vi "force_control_loop_1axis.vi"(0 "Force In":dbl[](array[numeric]), 5 "Goal Position IN":dbl[][](array[numeric]), 7 "Force Stimulus":dbl[](array[numeric])) -> (6 "Force Position Out":dbl[](array[numeric]), 15 "Last Error":dbl[](array[numeric]))   [LabVIEW 2013]
uses:
  <vilib>/Analysis/NI_AALBase.lvlib
  <vilib>/Analysis/baseanly.llb/Real A x B.vi
  <vilib>/Analysis/Matrix/NI_Matrix.lvlib
  <vilib>/Analysis/Matrix/Numeric/Conversions/Matrix To Array - RM.vi
  force_control_globals.vi
  <vilib>/Analysis/Matrix/Datatypes/RealMatrix.ctl
panel:
  out "Goal Position HOLD":dbl[][](array[numeric])
  out "Last dForce":dbl[](array[numeric])
  out "Inject Stimulus":bool
  out "Last Force":dbl[](array[numeric])
  in  "Accel Transform":T1
  out "Last Ki":dbl[](array[numeric])
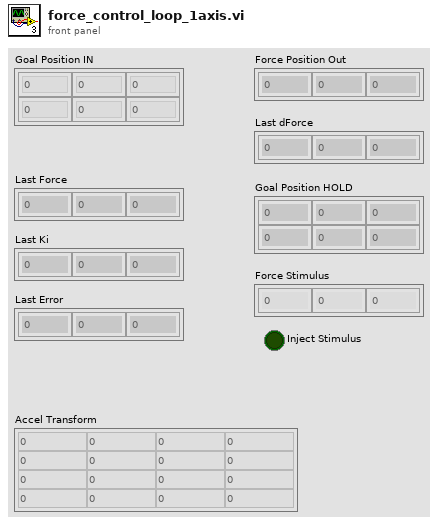
[diagram p1: front panel]
types:
  T1 = typedef "NI_Matrix.lvlib/RealMatrix.ctl" = dbl[][]
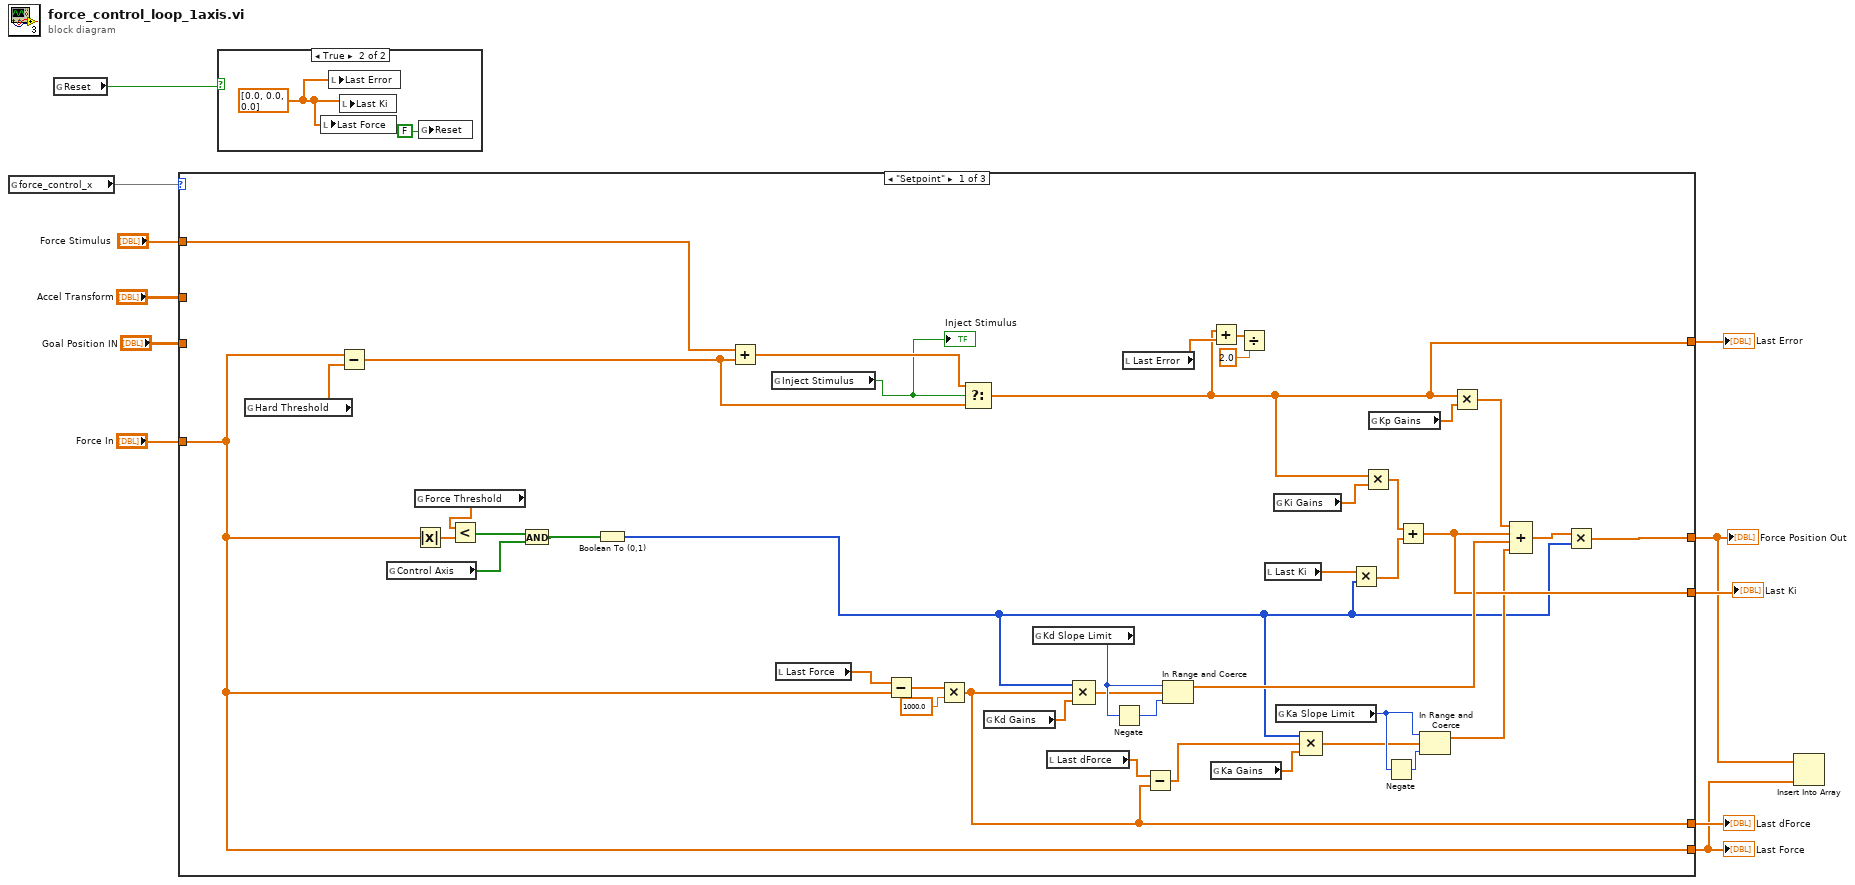
[diagram p0: block diagram]
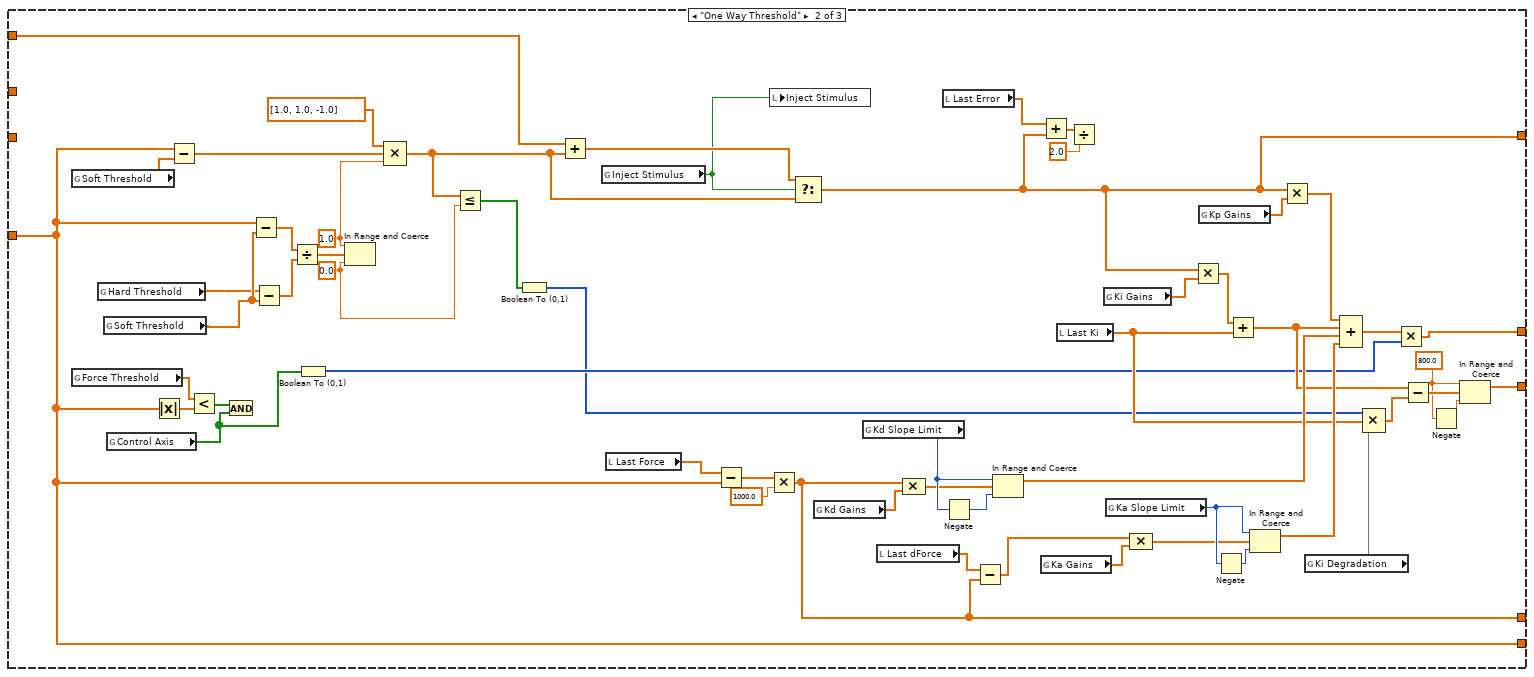
[diagram p3: hidden frame]
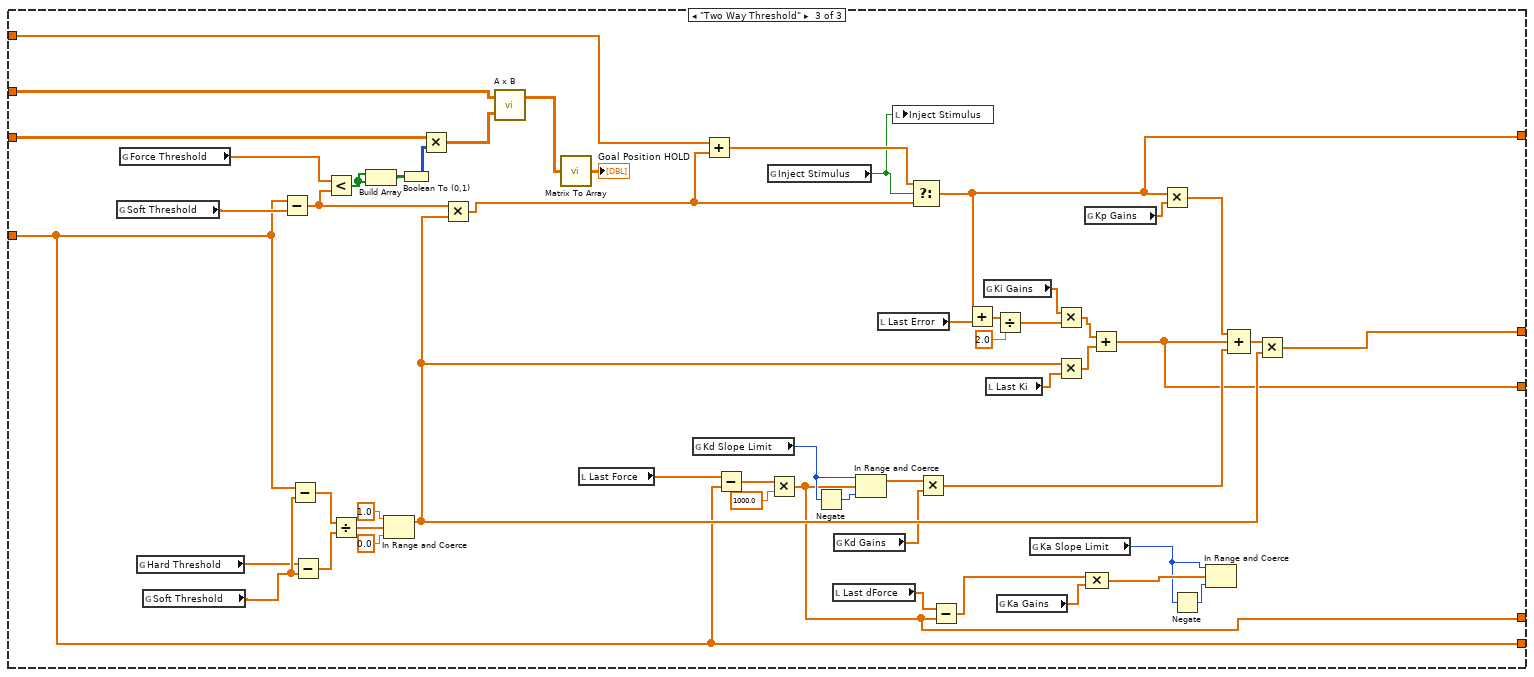
[diagram p4: hidden frame]
diagram:
  n1 = global read "force_control_globals.vi" "force_control_x"() -> (w10)
  n2 = global read "force_control_globals.vi" "Reset"() -> (w5:bool)
  n3 = case shown="\"Setpoint\"" w10 {
    tunnel: "Force In" -> [w34 w76 w112]
    tunnel: [w28 w57 w109] -> w4
    tunnel: [w27 w71 w147] -> w7
    tunnel: [w30 w59 w145] -> w2
    tunnel: "Accel Transform" -> [_ _ w132]
    tunnel: "Force Stimulus" -> [w41 w98 w120]
    tunnel: [w34 w76 w112] -> w1
    tunnel: "Goal Position IN" -> [_ _ w118]
    tunnel: [w22 w87 w111] -> w6
    frame "Setpoint" {
      n4 = global read "force_control_globals.vi" "Hard Threshold"() -> (w39:sgl[])
      n5 = Subtract(x=w34, y=w39) -> (x-y=w36:dbl[])
      n6 = global read "force_control_globals.vi" "Control Axis"() -> (w13:bool[])
      n7 = global read "force_control_globals.vi" "Force Threshold"() -> (w16:sgl[])
      n8 = Absolute Value(x=w34) -> (abs(x)=w52:dbl[])
      n9 = Less?(x=w16, y=w52) -> (x < y?=w14:bool[])
      n10 = And(x=w14, y=w13) -> (x .and. y?=w15:bool[])
      n11 = Boolean To (0,1)(Boolean=w15) -> (0, 1=w12:i16[])
      n12 = Add(x=w41, y=w36) -> (x+y=w51:dbl[])
      n13 = global read "force_control_globals.vi" "Inject Stimulus"() -> (w37:bool)
      "Inject Stimulus" <- w37
      n14 = local read "Last Force"() -> (w47:dbl[])
      n15 = Subtract(x=w47, y=w34) -> (x-y=w49:dbl[])
      n16 = Multiply(x=w49, y=1000.0) -> (x*y=w22:dbl[])
      n17 = Select(t=w51, s=w37, f=w36) -> (s? t:f=w27:dbl[])
      n18 = global read "force_control_globals.vi" "Kd Gains"() -> (w38:sgl[])
      n19 = global read "force_control_globals.vi" "Kd Slope Limit"() -> (w33:i32)
      n20 = local read "Last dForce"() -> (w23:dbl[])
      n21 = Compound Arithmetic op=MULTIPLY(w12, w22, w38) -> (w32:dbl[])
      n22 = Negate(x=w33) -> (-x=w46:i32)
      n23 = local read "Last Error"() -> (w43:dbl[])
      n24 = Subtract(x=w23, y=w22) -> (x-y=w21:dbl[])
      n25 = In Range and Coerce(upper limit=w33, x=w32, lower limit=w46) -> (coerced(x)=w31:dbl[])  [unwired: 1 out]
      n26 = Add(x=w27, y=w43) -> (x+y=w44:dbl[])
      n27 = global read "force_control_globals.vi" "Ka Gains"() -> (w24:sgl[])
      n28 = Divide(x=w44, y=2.0) -> ()  [unwired: 1 out]
      n29 = local read "Last Ki"() -> (w25:dbl[])
      n30 = global read "force_control_globals.vi" "Ki Gains"() -> (w35:sgl[])
      n31 = global read "force_control_globals.vi" "Ka Slope Limit"() -> (w19:i32)
      n32 = Compound Arithmetic op=MULTIPLY(w12, w21, w24) -> (w18:dbl[])
      n33 = Multiply(x=w25, y=w12) -> (x*y=w26:dbl[])
      n34 = Multiply(x=w27, y=w35) -> (x*y=w42:dbl[])
      n35 = global read "force_control_globals.vi" "Kp Gains"() -> (w40:sgl[])
      n36 = Negate(x=w19) -> (-x=w20:i32)
      n37 = Add(x=w42, y=w26) -> (x+y=w28:dbl[])
      n38 = In Range and Coerce(upper limit=w19, x=w18, lower limit=w20) -> (coerced(x)=w17:dbl[])  [unwired: 1 out]
      n39 = Multiply(x=w27, y=w40) -> (x*y=w50:dbl[])
      n40 = Compound Arithmetic op=ADD(w50, w28, w31, w17) -> (w29:dbl[])
      n41 = Multiply(x=w29, y=w12) -> (x*y=w30:dbl[])
    }
    frame "One Way Threshold" {
      w54 = 800.0
      w72 = 1.0 ("upper limit")
      w62 = 0.0 ("lower limit")
      n42 = global read "force_control_globals.vi" "Soft Threshold"() -> (w96:sgl[])
      n43 = global read "force_control_globals.vi" "Force Threshold"() -> (w81:sgl[])
      n44 = global read "force_control_globals.vi" "Hard Threshold"() -> (w78:sgl[])
      n45 = global read "force_control_globals.vi" "Soft Threshold"() -> (w79:sgl[])
      n46 = global read "force_control_globals.vi" "Control Axis"() -> (w63:bool[])
      n47 = Absolute Value(x=w76) -> (abs(x)=w108:dbl[])
      n48 = Subtract(x=w76, y=w96) -> (x-y=w75:dbl[])
      n49 = Less?(x=w81, y=w108) -> (x < y?=w70:bool[])
      n50 = And(x=w70, y=w63) -> ()  [unwired: 1 out]
      n51 = Subtract(x=w76, y=w79) -> (x-y=w77:dbl[])
      n52 = Subtract(x=w78, y=w79) -> (x-y=w64:sgl[])
      n53 = Divide(x=w77, y=w64) -> (x/y=w80:dbl[])
      n54 = Boolean To (0,1)(Boolean=w63) -> (0, 1=w61:i16[])
      n55 = In Range and Coerce(upper limit=w72, x=w80, lower limit=w62) -> ()  [unwired: 2 out]
      n56 = Compound Arithmetic op=MULTIPLY(dbl[] [1.0, 1.0, -1.0], w75, w72) -> (w66:dbl[])
      n57 = Less Or Equal?(x=w66, y=w62) -> (x <= y?=w65:bool[])
      n58 = Boolean To (0,1)(Boolean=w65) -> (0, 1=w60:i16[])
      n59 = Add(x=w98, y=w66) -> (x+y=w107:dbl[])
      n60 = global read "force_control_globals.vi" "Inject Stimulus"() -> (w74:bool)
      n61 = local read "Last Force"() -> (w103:dbl[])
      n62 = Subtract(x=w103, y=w76) -> (x-y=w105:dbl[])
      n63 = Multiply(x=w105, y=1000.0) -> (x*y=w87:dbl[])
      n64 = local write "Inject Stimulus"(w74) -> ()
      n65 = Select(t=w107, s=w74, f=w66) -> (s? t:f=w71:dbl[])
      n66 = global read "force_control_globals.vi" "Kd Gains"() -> (w95:sgl[])
      n67 = global read "force_control_globals.vi" "Kd Slope Limit"() -> (w93:i32)
      n68 = local read "Last dForce"() -> (w88:dbl[])
      n69 = Compound Arithmetic op=MULTIPLY(w87, w95) -> (w92:dbl[])
      n70 = local read "Last Error"() -> (w73:dbl[])
      n71 = Negate(x=w93) -> (-x=w102:i32)
      n72 = Subtract(x=w88, y=w87) -> (x-y=w86:dbl[])
      n73 = In Range and Coerce(upper limit=w93, x=w92, lower limit=w102) -> (coerced(x)=w91:dbl[])  [unwired: 1 out]
      n74 = Add(x=w73, y=w71) -> (x+y=w100:dbl[])
      n75 = global read "force_control_globals.vi" "Ka Gains"() -> (w89:sgl[])
      n76 = local read "Last Ki"() -> (w68:dbl[])
      n77 = Divide(x=w100, y=2.0) -> ()  [unwired: 1 out]
      n78 = global read "force_control_globals.vi" "Ki Gains"() -> (w94:sgl[])
      n79 = global read "force_control_globals.vi" "Ka Slope Limit"() -> (w84:i32)
      n80 = Compound Arithmetic op=MULTIPLY(w86, w89) -> (w83:dbl[])
      n81 = Multiply(x=w71, y=w94) -> (x*y=w99:dbl[])
      n82 = global read "force_control_globals.vi" "Kp Gains"() -> (w97:sgl[])
      n83 = Negate(x=w84) -> (-x=w85:i32)
      n84 = Add(x=w99, y=w68) -> (x+y=w69:dbl[])
      n85 = In Range and Coerce(upper limit=w84, x=w83, lower limit=w85) -> (coerced(x)=w82:dbl[])  [unwired: 1 out]
      n86 = Multiply(x=w71, y=w97) -> (x*y=w106:dbl[])
      n87 = global read "force_control_globals.vi" "Ki Degradation"() -> (w58)
      n88 = Compound Arithmetic op=ADD(w106, w69, w91, w82) -> (w90:dbl[])
      n89 = Compound Arithmetic op=MULTIPLY(w60, w68, w58) -> (w67:dbl[])
      n90 = Multiply(x=w90, y=w61) -> (x*y=w59:dbl[])
      n91 = Subtract(x=w69, y=w67) -> (x-y=w56:dbl[])
      n92 = Negate(x=w54) -> (-x=w55:dbl)
      n93 = In Range and Coerce(upper limit=w54, x=w56, lower limit=w55) -> (coerced(x)=w57:dbl[])  [unwired: 1 out]
    }
    frame "Two Way Threshold" {
      n94 = global read "force_control_globals.vi" "Soft Threshold"() -> (w122:sgl[])
      n95 = global read "force_control_globals.vi" "Force Threshold"() -> (w121:sgl[])
      n96 = global read "force_control_globals.vi" "Hard Threshold"() -> (w123:sgl[])
      n97 = global read "force_control_globals.vi" "Soft Threshold"() -> (w124:sgl[])
      n98 = Subtract(x=w112, y=w122) -> (x-y=w136:dbl[])
      n99 = Subtract(x=w112, y=w124) -> (x-y=w141:dbl[])
      n100 = Subtract(x=w123, y=w124) -> (x-y=w140:sgl[])
      n101 = Less?(x=w121, y=w136) -> (x < y?=w135:bool[])
      n102 = Divide(x=w141, y=w140) -> (x/y=w139:dbl[])
      n103 = Build Array(w135, w135) -> (w133:bool[][])
      n104 = In Range and Coerce(upper limit=1.0, x=w139, lower limit=0.0) -> (coerced(x)=w137:dbl[])  [unwired: 1 out]
      n105 = Boolean To (0,1)(Boolean=w133) -> (0, 1=w134:i16[][])
      n106 = Multiply(x=w118, y=w134) -> (x*y=w131:dbl[][])
      n107 = Multiply(x=w136, y=w137) -> (x*y=w138:dbl[])
      n108 = call-poly <vilib>:"A x B.vi"("B"=w131, "A"=w132) -> ("A x B"=w129:T1)  [unwired: 1 out]
      n109 = call-poly <vilib>:"Matrix To Array.vi"("Real Matrix"=w129) -> ("Real 2D Array"=→"Goal Position HOLD":dbl[][])
      n110 = local read "Last Force"() -> (w156:dbl[])
      n111 = global read "force_control_globals.vi" "Kd Slope Limit"() -> (w125:i32)
      n112 = Add(x=w120, y=w138) -> (x+y=w161:dbl[])
      n113 = Subtract(x=w156, y=w112) -> (x-y=w158:dbl[])
      n114 = global read "force_control_globals.vi" "Inject Stimulus"() -> (w119:bool)
      n115 = Multiply(x=w158, y=1000.0) -> (x*y=w111:dbl[])
      n116 = Negate(x=w125) -> (-x=w155:i32)
      n117 = local read "Last dForce"() -> (w116:dbl[])
      n118 = global read "force_control_globals.vi" "Kd Gains"() -> (w126:sgl[])
      n119 = In Range and Coerce(upper limit=w125, x=w111, lower limit=w155) -> (coerced(x)=w154:dbl[])  [unwired: 1 out]
      n120 = local read "Last Error"() -> (w149:dbl[])
      n121 = local write "Inject Stimulus"(w119) -> ()
      n122 = Select(t=w161, s=w119, f=w138) -> (s? t:f=w147:dbl[])
      n123 = Multiply(x=w154, y=w126) -> (x*y=w159:dbl[])
      n124 = Subtract(x=w116, y=w111) -> (x-y=w115:dbl[])
      n125 = Add(x=w147, y=w149) -> (x+y=w150:dbl[])
      n126 = global read "force_control_globals.vi" "Ki Gains"() -> (w127:sgl[])
      n127 = local read "Last Ki"() -> (w152:dbl[])
      n128 = Divide(x=w150, y=2.0) -> (x/y=w148:dbl[])
      n129 = global read "force_control_globals.vi" "Ka Gains"() -> (w117:sgl[])
      n130 = global read "force_control_globals.vi" "Ka Slope Limit"() -> (w110:i32)
      n131 = Multiply(x=w127, y=w148) -> (x*y=w144:dbl[])
      n132 = Multiply(x=w137, y=w152) -> (x*y=w153:dbl[])
      n133 = global read "force_control_globals.vi" "Kp Gains"() -> (w128:sgl[])
      n134 = Compound Arithmetic op=MULTIPLY(w115, w117) -> (w113:dbl[])
      n135 = Add(x=w144, y=w153) -> (x+y=w109:dbl[])
      n136 = Multiply(x=w147, y=w128) -> (x*y=w160:dbl[])
      n137 = Negate(x=w110) -> (-x=w114:i32)
      n138 = In Range and Coerce(upper limit=w110, x=w113, lower limit=w114) -> ()  [unwired: 2 out]
      n139 = Compound Arithmetic op=ADD(w160, w109, w159) -> (w146:dbl[])
      n140 = Multiply(x=w146, y=w137) -> (x*y=w145:dbl[])
    }
  }
  "Last Error" <- w7
  "Last Ki" <- w4
  "Force Position Out" <- w2
  "Last Force" <- w1
  "Last dForce" <- w6
  n141 = case shown="True" w5 {
    frame False {
    }
    frame True {
      w163 = dbl[] [0.0, 0.0, 0.0]
      n142 = local write "Last Force"(w163) -> ()
      n143 = local write "Last Error"(w163) -> ()
      n144 = local write "Last Ki"(w163) -> ()
      n145 = global write "force_control_globals.vi" "Reset"(FALSE) -> ()
    }
  }
  n146 = Insert Into Array(array=w2, new element=w1) -> ()  [unwired: 1 in, 1 out]
